vi "Callib.vi"(11 "VISA resource name":refnum<visa-resource-name>="COM7") -> (2 "read string":string)   [LabVIEW 2017]
uses:
  controls/#typedef_Queue Cmd.ctl
panel:
  in  "Callib Button":bool
  out "error out":errorcluster
  in  "error in (no error)":errorcluster
  in  "stop":bool
  in  "Get ID Button":bool
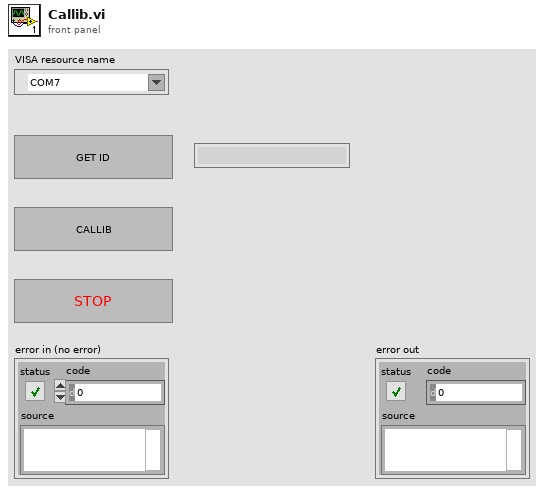
[diagram p1: front panel]
types:
  T1 = typedef "#typedef_Queue Cmd.ctl" = enum16{"Get ID", "Callib", "Go to", "Exit"}
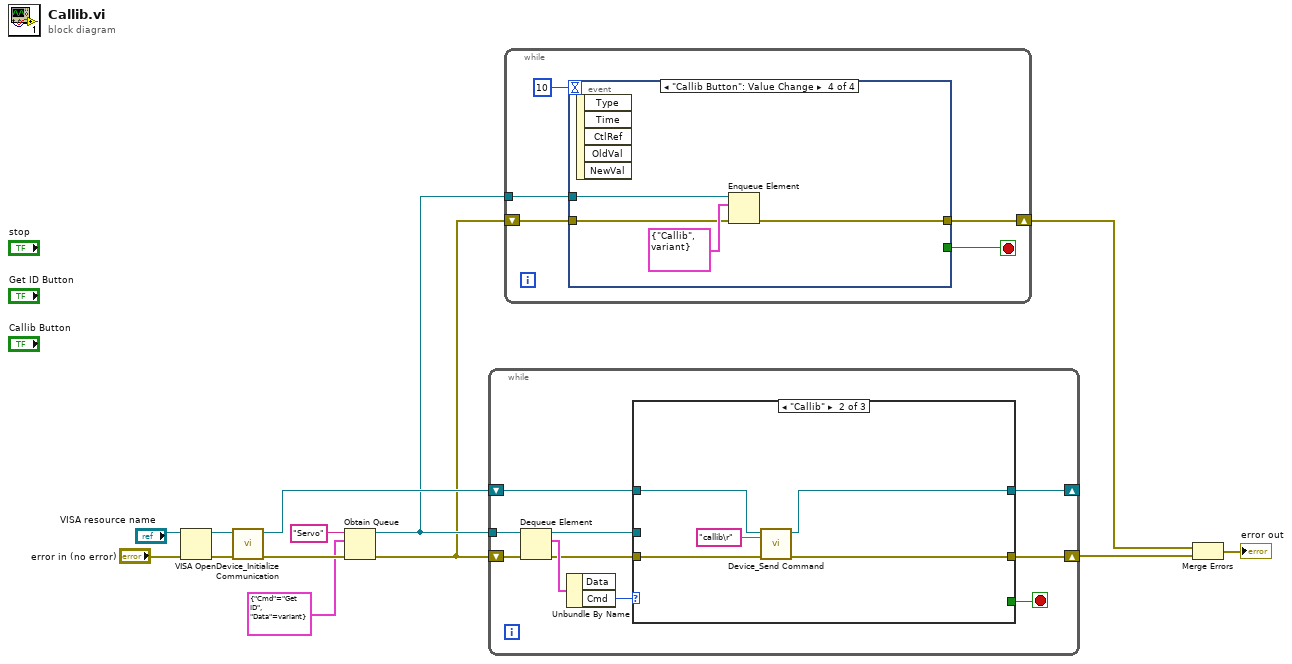
[diagram p0: block diagram]
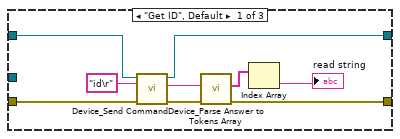
[diagram p2: hidden frame]
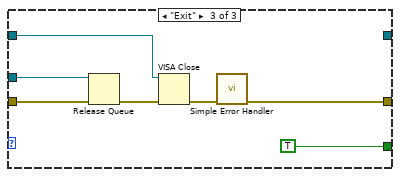
[diagram p3: hidden frame]
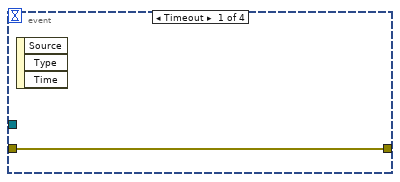
[diagram p4: hidden frame]
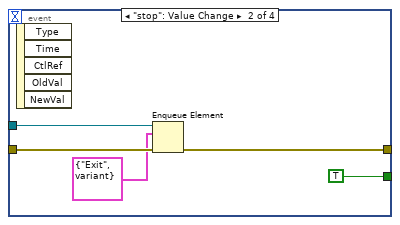
[diagram p5: hidden frame]
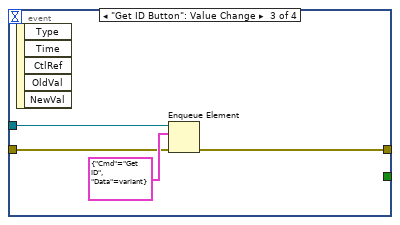
[diagram p6: hidden frame]
diagram:
  n1 = VISA Open(error in (no error)="error in (no error)", VISA resource name="VISA resource name") -> (VISA resource name=w12:refnum<visa-resource-name>, error out=w11:errorcluster)  [unwired: 3 in]
  n2 = call "Device_Initialize Communication.vi"("error in (no error)"=w11, "VISA Refnum in"=w12) -> ("error out"=w9:errorcluster, "VISA Refnum out"=w8:refnum<visa-resource-name>)  [unwired: 8 in]
  n3 = Obtain Queue(name (unnamed)="Servo", element data type=cluster{"Cmd":T1, "Data":variant} {"Cmd"=enum."Get ID", "Data"=variant} ("Queue Msg"), error in (no error)=w9) -> (queue out=w5:refnum<queue>, error out=w4:errorcluster)  [unwired: 2 in, 1 out]
  n4 = while {
    shift-right: [w14] -> _
    shift-left: w8 -> [w15]
    tunnel: w5 -> [w22]
    shift-right: [w17] -> w3
    shift-left: w4 -> [w23]
    stop <- w16 stop-if-true
    n5 = Dequeue Element(queue=w22, error in (no error)=w23) -> (queue out=w18:refnum<queue>, element=w21:cluster{"Cmd":T1, "Data":variant}, error out=w19:errorcluster)  [unwired: 1 in, 1 out]
    n6 = Unbundle By Name(w21) -> ("Cmd"=w20:T1)  [unwired: 1 out]
    n7 = case shown="\"Callib\"" w20 {
      tunnel: w19 -> [w30 w35 w44]
      tunnel: w18 -> [_ _ w43]
      tunnel: [w27 w33 w38] -> w17
      tunnel: [_ _ TRUE] -> w16
      tunnel: w15 -> [w31 w36 w40]
      tunnel: [w29 w34 _] -> w14
      frame "Get ID", Default {
        n8 = call "Device_Send Command.vi"("error in (no error)"=w30, "write string"="id\r", "VISA Refnum in"=w31) -> ("error out"=w28:errorcluster, "read buffer"=w26:string, "VISA Refnum out"=w29:refnum<visa-resource-name>)  [unwired: 6 in]
        n9 = call "Device_Parse Answer to Tokens Array.vi"("error in (no error)"=w28, "Answer"=w26) -> ("error out"=w27:errorcluster, "Tokens Array"=w25:string[])  [unwired: 8 in]
        n10 = Index Array(array=w25) -> (element=→"read string":string)  [unwired: 1 in]
      }
      frame "Callib" {
        n11 = call "Device_Send Command.vi"("error in (no error)"=w35, "write string"="callib\r", "VISA Refnum in"=w36) -> ("error out"=w33:errorcluster, "VISA Refnum out"=w34:refnum<visa-resource-name>)  [unwired: 6 in, 1 out]
      }
      frame "Exit" {
        n12 = Release Queue(queue=w43, error in (no error)=w44) -> (error out=w39:errorcluster)  [unwired: 1 in, 2 out]
        n13 = VISA Close(VISA resource name=w40, error in (no error)=w39) -> (error out=w41:errorcluster)
        n14 = call <vilib>:"Simple Error Handler.vi"("error in (no error)"=w41) -> ("error out"=w38:errorcluster)  [unwired: 4 in, 4 out]
      }
    }
  }
  n15 = while {
    tunnel: w5 -> [w49]
    shift-right: [w47] -> w2
    shift-left: w4 -> [w48]
    stop <- w46 stop-if-true
    n16 = event shown="[3] \"Callib Button\": Value Change" {
      selector: _ -> [_ _ _ _]
      dyn-events: _ -> [_ _ _ _]
      timeout: 10 -> [_ _ _ _]
      tunnel: w49 -> [_ w52 w57 w61]
      tunnel: w48 -> [w50 w55 w58 w62]
      tunnel: [w50 w54 w56 w60] -> w47
      tunnel: [_ TRUE _ _] -> w46
      event Timeout {
        n17 = event-data() -> ()  [unwired: 1 in, 3 out]
      }
      event "stop": Value Change {
        n18 = event-data() -> ()  [unwired: 1 in, 5 out]
        n19 = Enqueue Element(queue=w52, element=cluster{"Cmd":T1, "Data":variant} {"Cmd"=enum."Exit", "Data"=variant} ("Queue Msg"), error in (no error)=w55) -> (error out=w54:errorcluster)  [unwired: 1 in, 2 out]
      }
      event "Get ID Button": Value Change {
        n20 = event-data() -> ()  [unwired: 1 in, 5 out]
        n21 = Enqueue Element(queue=w57, element=cluster{"Cmd":T1, "Data":variant} {"Cmd"=enum."Get ID", "Data"=variant} ("Queue Msg"), error in (no error)=w58) -> (error out=w56:errorcluster)  [unwired: 1 in, 2 out]
      }
      event "Callib Button": Value Change {
        n22 = event-data() -> ()  [unwired: 1 in, 5 out]
        n23 = Enqueue Element(queue=w61, element=cluster{"Cmd":T1, "Data":variant} {"Cmd"=enum."Callib", "Data"=variant} ("Queue Msg"), error in (no error)=w62) -> (error out=w60:errorcluster)  [unwired: 1 in, 2 out]
      }
    }
  }
  n24 = Merge Errors(w2, w3) -> (→"error out":errorcluster)
